vi "LoadObject.vi"(8 "No Error":errorcluster, 11 "Shared Object File":string) -> (0 "Error Out":errorcluster, 3 "Handle [SDL_SharedObject *]":T1 format="%.0x")   [LabVIEW 2026, in "SDL3.lvlib" / "LoadSO.lvlib"]
doc: "<B>Summary</B>\nDynamically load a shared object."
uses:
  LoadSO.lvlib
  <vilib>/Utility/error.llb/Error Cluster From Error Code.vi
  Error/Error.lvlib
  Lib/SDL3.dll
  SDL_SharedObject--pointer.ctl
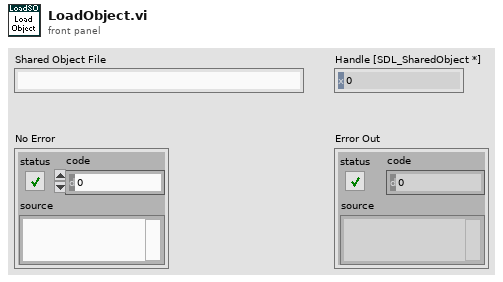
[diagram p1: front panel]
types:
  T1 = typedef "SDL3.lvlib/LoadSO.lvlib/SDL_SharedObject--pointer.ctl" = i64
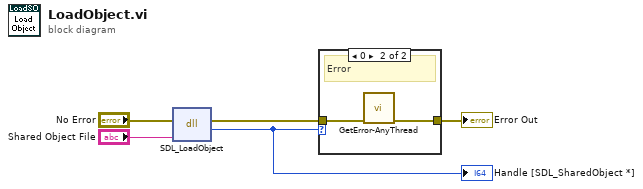
[diagram p0: block diagram]
diagram:
  n1 = dll-call lib="C:/Users/saukko/Dev/LV-SDL3/Sources/SDL3/Lib/SDL3.*" fn="SDL_LoadObject"(error in="No Error", "sofile"="Shared Object File") -> (error out=w2:errorcluster, "return type"=w4:i64)  [unwired: 3 in, 1 out]
  "Handle [SDL_SharedObject *]" <- w4
  n2 = case shown="0" w4 {
    tunnel: w2 -> [w6 w8]
    tunnel: [w6 w7] -> w3
    frame Default {
      # "Ok"
    }
    frame 0 {
      # "Error"
      n3 = call "GetError-AnyThread.vi"("No Error"=w8) -> ("Error Out"=w7:errorcluster)  [unwired: 10 in]
    }
  }
  "Error Out" <- w3
